vi "get_position.vi"(8 "error in (no error)":errorcluster, 11 "ESP301_via_TCPIP in":refnum<class "ESP301_via_TCPIP.lvclass">) -> (0 "error out":errorcluster, 2 "last position":dbl, 3 "ESP301_via_TCPIP out":refnum<class "ESP301_via_TCPIP.lvclass">)   [LabVIEW 2019, in "ESP301_via_TCPIP.lvclass"]
uses:
  ESP301_via_TCPIP.lvclass
  _delayStageBase/_delayStageBase.lvclass
panel:
  out "Numeric":i32
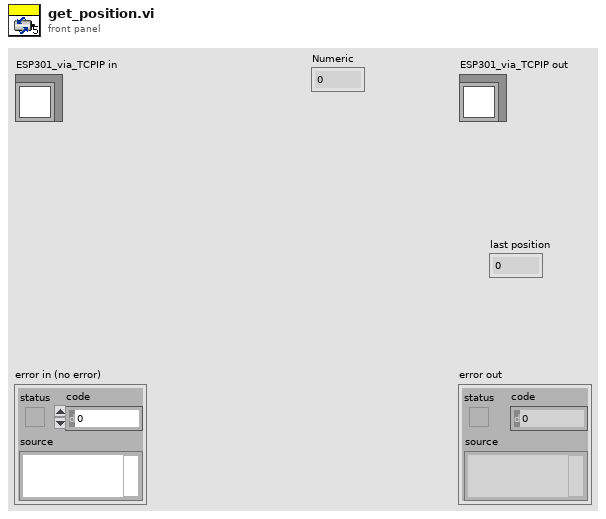
[diagram p1: front panel]
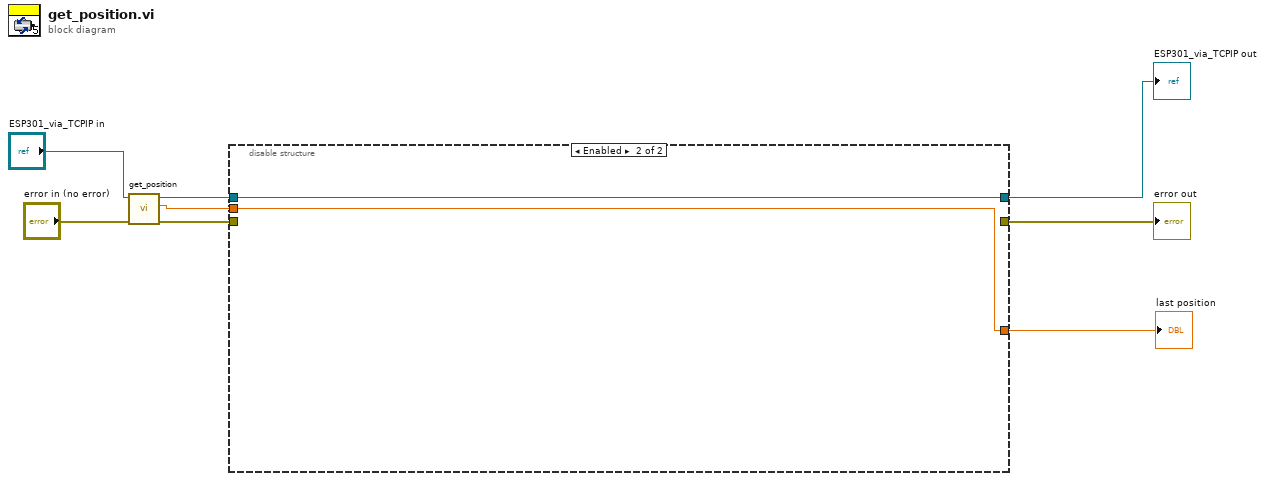
[diagram p0: block diagram]
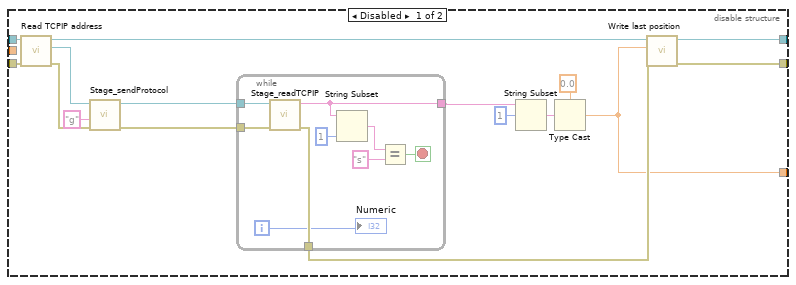
[diagram p2: hidden frame]
diagram:
  n1 = call-parent "get_position.vi"("error in (no error)"="error in (no error)", "_delayStageBase in"="ESP301_via_TCPIP in") -> ("error out"=w5:errorcluster, "last position"=w1:dbl, "_delayStageBase out"=w6:refnum<class "ESP301_via_TCPIP.lvclass">)  [unwired: 7 in]
  n2 = disable-structure shown="Enabled" {
    disable-tunnel: w6 -> [w24 w35]
    disable-tunnel: w5 -> [w23 _]
    disable-tunnel: [w11 w35] -> w4
    disable-tunnel: [w10 _] -> w3
    disable-tunnel: [w9 w34] -> w2
    disable-tunnel: w1 -> [_ w34]
    frame Disabled {
      n3 = call-dynamic "Read TCPIP address.vi"("error in (no error)"=w23, "ESP301_via_TCPIP in"=w24) -> ("error out"=w21:errorcluster, "TCPIP address"=w22:refnum<k5>, "ESP301_via_TCPIP out"=w13:refnum<class "ESP301_via_TCPIP.lvclass">)  [unwired: 7 in]
      n4 = call "Stage_sendProtocol.vi"("error in (no error)"=w21, "command"="g", "TCP Network Connection in"=w22) -> ("error out"=w18:errorcluster, "TCP Network Connection out"=w19:refnum<k5>)  [unwired: 7 in]
      n5 = while {
        tunnel: w19 -> [w33]
        tunnel: [w30] -> w14
        tunnel: w18 -> [w27]
        tunnel: [w26] -> w12
        i -> [w25]
        stop <- w31 stop-if-true
        n6 = call "Stage_readTCPIP.vi"("error in (no error)"=w27, "TCP Network Connection in"=w33) -> ("error out"=w26:errorcluster, "data out"=w30:string)  [unwired: 8 in]
        n7 = String Subset(string=w30, length (rest)=1 ("offset (0)")) -> (substring=w28:string)  [unwired: 1 in]
        n8 = Equal?(x=w28, y="s") -> (x = y?=w31:bool)
        "Numeric" <- w25
      }
      n9 = String Subset(string=w14, offset (0)=1) -> (substring=w16:string)  [unwired: 1 in]
      n10 = Type Cast(type=0.0, x=w16) -> (*(type *) &x=w9:dbl)
      n11 = call-dynamic "Write last position.vi"("error in (no error)"=w12, "last position"=w9, "_delayStageBase in"=w13) -> ("error out"=w10:errorcluster, "_delayStageBase out"=w11:refnum<class "ESP301_via_TCPIP.lvclass">)  [unwired: 7 in]
    }
    frame Enabled {
    }
  }
  "error out" <- w3
  "ESP301_via_TCPIP out" <- w4
  "last position" <- w2
